vi "String to WSTRING Byte Stream.vi"(8 "error in (no error)":errorcluster, 10 "Value":string) -> (0 "error out":errorcluster, 2 "Byte Stream":u8[](array[numeric]))   [LabVIEW 2018, in "TwinCAT ADS.lvclass"]
uses:
  TwinCAT ADS.lvclass
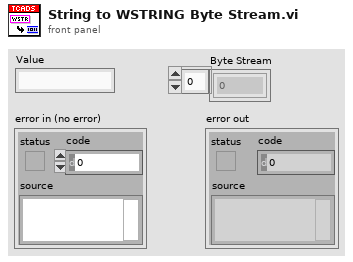
[diagram p1: front panel]
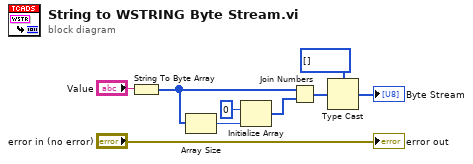
[diagram p0: block diagram]
diagram:
  n1 = String To Byte Array(string="Value") -> (unsigned byte array=w4:u8[])
  n2 = Array Size(array=w4) -> (size(s)=w8:i32)
  n3 = Initialize Array(u8 0 ("dimension size"), w8) -> (w7:u8[])
  n4 = Join Numbers(hi=w4, lo=w7) -> ((hi.lo)=w5:u16[])
  n5 = Type Cast(type=u8[] [] ("initialized array"), x=w5) -> (*(type *) &x=→"Byte Stream":u8[])
  "error out" <- "error in (no error)"
